vi "Close Web Client.vi"(8 "error in (no error)":errorcluster, 11 "Web Client in":refnum<class "Web Client.lvclass">) -> (0 "error out":errorcluster)   [LabVIEW 2018, in "Collaborator.lvlib" / "Web Client.lvclass"]
uses:
  Web Client.lvclass
  Web Client.lvclass/Web Client.ctl
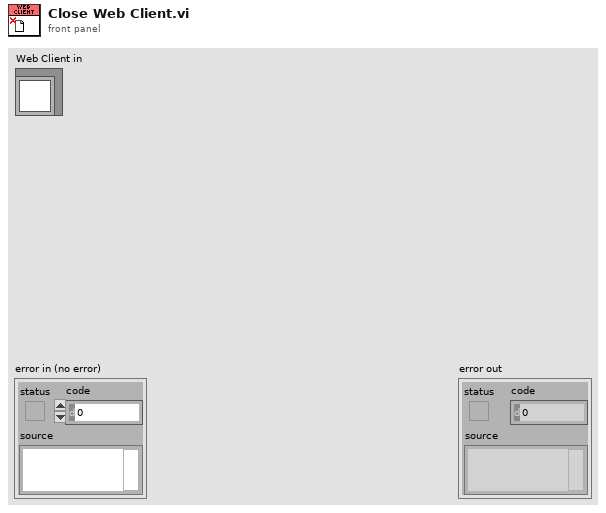
[diagram p1: front panel]
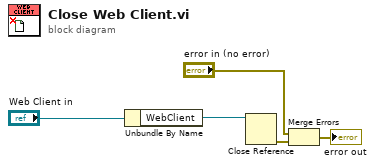
[diagram p0: block diagram]
diagram:
  n1 = Unbundle By Name("Web Client in") -> ("WebClient"=w3:refnum<k24>)
  n2 = Close Reference(reference=w3) -> (error out=w1:errorcluster)  [unwired: 1 in]
  n3 = Merge Errors("error in (no error)", w1) -> (→"error out":errorcluster)
